vi "Do Get Reference.vi"(8 "error in (no error)":errorcluster, 10 "Get Reference Argument":T2, 11 "Data Cluster in":T1) -> (0 "error out":errorcluster, 3 "Data Cluster out":T1)   [LabVIEW 2020, in "G-AI Core.lvlib"]
uses:
  G-AI Core.lvlib
  Get Reference (Reply Payload)--cluster.ctl
  Module Data--cluster.ctl
  Get Reference Argument--cluster.ctl
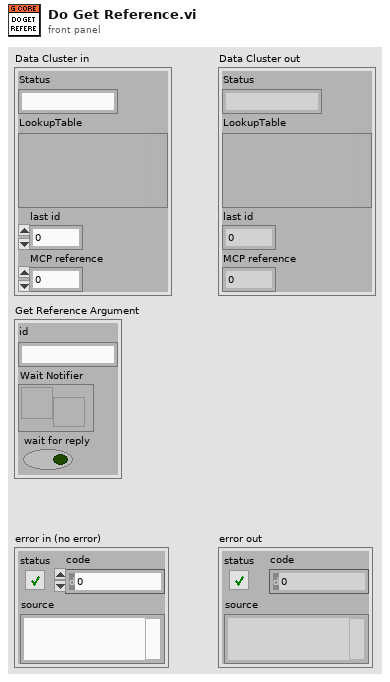
[diagram p1: front panel]
types:
  T1 = typedef "G-AI Core.lvlib/Module Data--cluster.ctl" = cluster{"Status":string, "LookupTable":variant, "last id":i32, "MCP reference":i32}
  T2 = typedef "G-AI Core.lvlib/Get Reference Argument--cluster.ctl" = cluster{"id":string, "Wait Notifier":refnum<notifier>, "wait for reply":bool}
  T3 = typedef "G-AI Core.lvlib/Get Reference (Reply Payload)--cluster.ctl" = cluster{"reference":variant, "error":errorcluster}
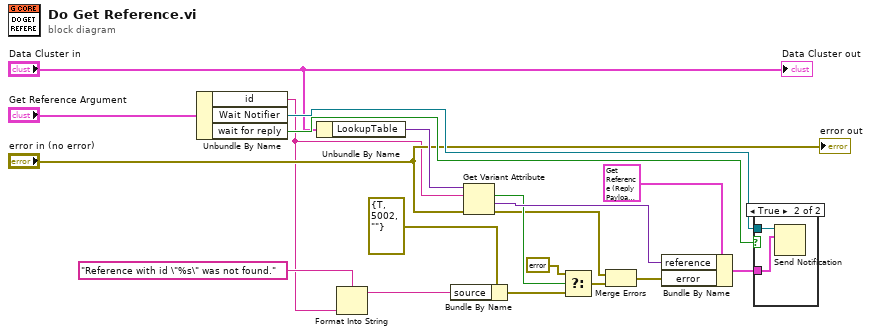
[diagram p0: block diagram]
diagram:
  n1 = Unbundle By Name("Get Reference Argument") -> ("id"=w4:string, "Wait Notifier"=w16:refnum<notifier>, "wait for reply"=w17:bool)
  n2 = Unbundle By Name("Data Cluster in") -> ("LookupTable"=w13:variant)
  n3 = Format Into String(format string="Reference with id \"%s\" was not found." ("source"), w4) -> (resulting string=w6:string)  [unwired: 2 in, 1 out]
  n4 = Bundle By Name(cluster=errorcluster {"status"=TRUE, "code"=5002, "source"=""} ("f"), "source"=w6) -> (w7:errorcluster)
  n5 = Get Variant Attribute(Variant=w13, name=w4, error in="error in (no error)") -> (found=w10:bool, value=w11:variant, error out=w1:errorcluster)  [unwired: 1 in, 1 out]
  n6 = Select(t=errorcluster {"status"=FALSE, "code"=0, "source"=""}, s=w10, f=w7) -> (s? t:f=w9:errorcluster)
  n7 = Merge Errors(w1, w9) -> (w3:errorcluster)
  n8 = Bundle By Name(cluster=T3 {"reference"=variant, "error"={"status"=FALSE, "code"=0, "source"=""}} ("Get Reference (Reply Payload)"), "reference"=w11, "error"=w3) -> (w18:T3)
  n9 = case "DQMH_FIRE_NOTIFIER" shown="True" w17 {
    tunnel: w16 -> [_ w21]
    tunnel: w18 -> [_ w20]
    frame False {
    }
    frame True {
      n10 = Send Notification(notification=w20, notifier=w21) -> ()  [unwired: 1 in, 2 out]
    }
  }
  "Data Cluster out" <- "Data Cluster in"
  "error out" <- "error in (no error)"
